vi "Get Network Settings.vi"(8 "error in":errorcluster, 11 "Item Ref in":T3 format="%.0x") -> (0 "error out":errorcluster, 2 "Network Settings":T1={"IP adress"="127.0.0.1", "RDB"={"Protocol"=enum."UDP", "Tx Port"=48191, "Rx Port"=48191, "Buffer Size"=204800, "Timeout"=10}, "SCP"={"Protocol"=enum."TCP", "Tx Port"=48191, "Rx Port"=48191, "Buffer Size"=204800, "Timeout"=10}}, 3 "Item Ref out":T3 format="%.0x")   [LabVIEW 2023, in "Vires VTD System Explorer.lvlib"]
uses:
  <vilib>/NI VeriStand/Custom Device API/Custom Device Item Ref.ctl
  Shared/Network Settings.ctl
  Shared/Protocol.ctl
  <vilib>/NI VeriStand/Custom Device Tools/Custom Device Utility Library/Search Direction.ctl
  Shared/Constants.vi
  <vilib>/NI VeriStand/Custom Device Tools/Custom Device Utility Library/NI VeriStand - Search for Item by GUID.vi
  <vilib>/NI VeriStand/Custom Device API/Get Item Property (Variant).vi
  Vires VTD System Explorer.lvlib
  Shared/Vires VTD Shared.lvlib
  <vilib>/NI VeriStand/Custom Device API/Custom Device API.lvlib
  <vilib>/NI VeriStand/Custom Device Tools/Custom Device Utility Library/Custom Device Utility Library.lvlib
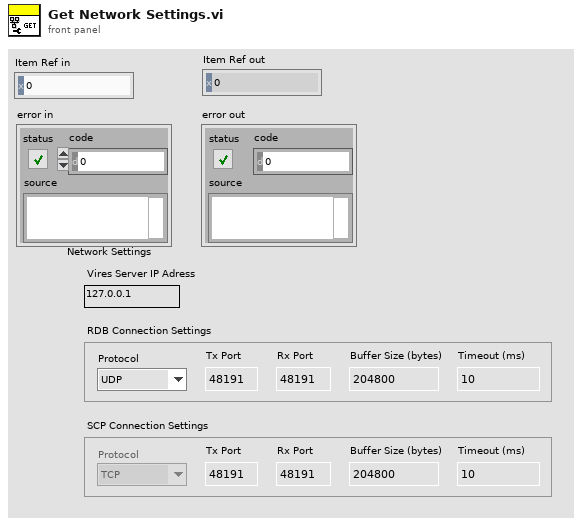
[diagram p1: front panel]
types:
  T1 = typedef "Vires VTD Shared.lvlib/Network Settings.ctl" = cluster{"IP adress":string, "RDB":cluster{"Protocol":T2, "Tx Port":u16, "Rx Port":u16, "Buffer Size":i32, "Timeout":u16}, "SCP":cluster{"Protocol":T2, "Tx Port":u16, "Rx Port":u16, "Buffer Size":i32, "Timeout":u16}}
  T2 = typedef "Vires VTD Shared.lvlib/Protocol.ctl" = enum16{"UDP", "TCP"}
  T3 = typedef "Custom Device API.lvlib/Custom Device Item Ref.ctl" = u64
  T4 = typedef "Custom Device API.lvlib/Custom Device Item Info.ctl" = cluster{"Name":string, "Is Channel":bool, "GUID":string, "Is Waveform":bool}
  T5 = typedef "Custom Device Utility Library.lvlib/Search Direction.ctl" = enum16{"Down", "Up"}
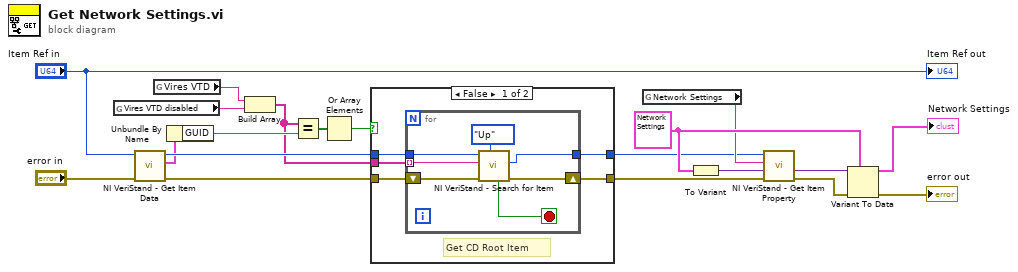
[diagram p0: block diagram]
diagram:
  w20 = T1 {"IP adress"="0.0.0.0", "RDB"={"Protocol"=enum."UDP", "Tx Port"=48191, "Rx Port"=48190, "Buffer Size"=204800, "Timeout"=10}, "SCP"={"Protocol"=enum."UDP", "Tx Port"=48179, "Rx Port"=48179, "Buffer Size"=204800, "Timeout"=10}} ("Network Settings")
  n1 = global read "Constants.vi" "Vires VTD disabled"() -> (w6:string)
  n2 = call <vilib>:"NI VeriStand - Get Item Data.vi"("error in (no error)"="error in", "Item Ref in"="Item Ref in") -> ("error out"=w10:errorcluster, "Item Info"=w7:T4, "Item Ref out"=w9:T3)  [unwired: 6 in, 1 out]
  n3 = global read "Constants.vi" "Vires VTD"() -> (w5:string)
  n4 = Unbundle By Name(w7) -> ("GUID"=w4:string)
  n5 = Build Array(w5, w6) -> (w1:string[])
  n6 = Equal?(x=w1, y=w4) -> (x = y?=w3:bool[])
  n7 = Or Array Elements(Boolean array=w3) -> (logical OR=w2:bool)
  n8 = case shown="False" w2 {
    tunnel: w10 -> [w25 w34]
    tunnel: [w24 w34] -> w13
    tunnel: [w23 w33] -> w12
    tunnel: w9 -> [w22 w33]
    tunnel: w1 -> [w21 _]
    frame False {
      # "Get CD Root Item"
      n9 = for {
        shift-right: [w30] -> w24
        shift-left: w25 -> [w31]
        tunnel: w21 -> [w27] mode=indexing
        tunnel: w22 -> [w28]
        tunnel: [w29] -> w23
        stop <- w26 stop-if-true
        n10 = call-poly <vilib>:"NI VeriStand - Search for Item.vi"("Direction (Down)"=Search_Direction."Up", "error in"=w31, "Item GUID"=w27, "Section Ref in"=w28) -> ("error out"=w30:errorcluster, "Item Ref"=w29:T3, "Found"=w26:bool)  [unwired: 4 in, 1 out]
      }
    }
    frame True {
      # "Item Ref in is CD Root Item"
    }
  }
  n11 = global read "Constants.vi" "Network Settings"() -> (w18:string)
  n12 = To Variant(anything=w20) -> (Variant=w17:variant)
  n13 = call-poly <vilib>:"NI VeriStand - Get Item Property.vi"("error in (no error)"=w13, "Default Value"=w17, "Property Name"=w18, "Item Ref in"=w12) -> ("error out"=w15:errorcluster, "Value"=w16:variant)  [unwired: 4 in, 2 out]
  n14 = Variant To Data(error in=w15, type=w20, Variant=w16) -> (data=→"Network Settings":T1, error out=→"error out":errorcluster)
  "Item Ref out" <- "Item Ref in"
